vi "InsertDataTo2DListCtrl.vi"(10 "arr data":string[][](array[string]), 11 "multiple list in":refnum<vi>) -> (3 "multiple list out":refnum<vi>)   [LabVIEW 2018, in "Library-Ctrl.lvlib"]
uses:
  Library-Ctrl.lvlib
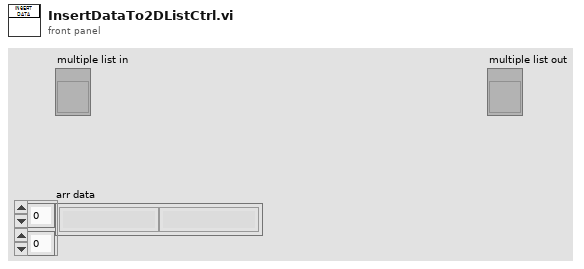
[diagram p1: front panel]
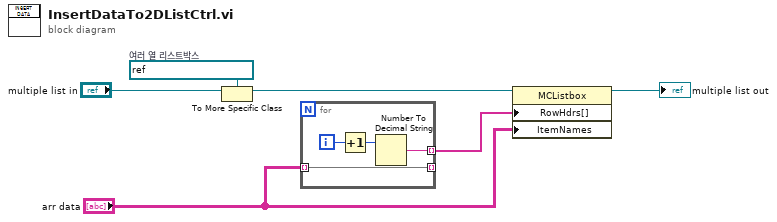
[diagram p0: block diagram]
diagram:
  w3 = refnum<vi> refnum  # 여러 열 리스트박스
  n1 = To More Specific Class(target class=w3, reference="multiple list in") -> (specific class reference=w1:refnum<vi>)  [unwired: 1 in, 1 out]
  n2 = for {
    tunnel: [w8] -> w4 mode=indexing
    tunnel: [w7] -> _ mode=indexing
    tunnel: "arr data" -> [w7] mode=indexing
    i -> [w10]
    n3 = Increment(x=w10) -> (x+1=w9:i32)
    n4 = Number To Decimal String(number=w9) -> (decimal integer string=w8:string)  [unwired: 1 in]
  }
  n5 = property class="MCListbox"(reference=w1, "RowHdrs[]"=w4, "ItemNames"="arr data") -> (reference out=→"multiple list out":refnum<vi>)  [unwired: 1 in, 1 out]
